vi "sCMOS_init_merFISH.vi"(4 "error in":errorcluster, 5 "Start acquisition":bool, 6 "N Frames":i32, 7 "handle":u32) -> (0 "error out":errorcluster {"code" format="%.0x"})   [LabVIEW 2015]
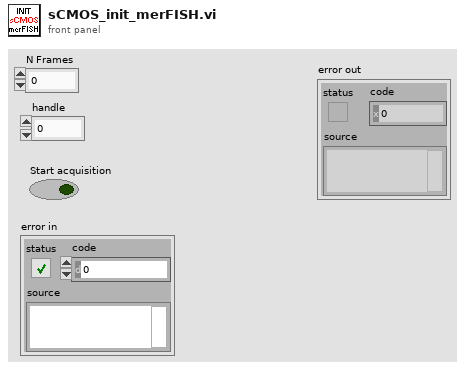
[diagram p1: front panel]
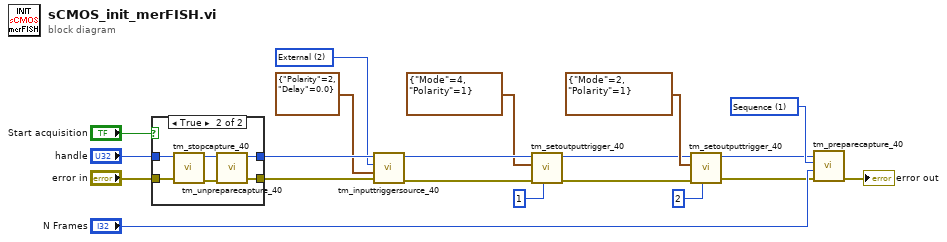
[diagram p0: block diagram]
diagram:
  w12 = 2 items=["Internal"=1, "External"=2, "Software"=3, "Master Pulse"=4] ("Source")
  w15 = 1 items=["Snap", "Sequence"] ("Capture mode")
  n1 = case shown="True" "Start acquisition" {
    tunnel: "error in" -> [w22 w28]
    tunnel: [w22 w24] -> w13
    tunnel: "handle" -> [w21 w27]
    tunnel: [w21 w23] -> w14
    frame False {
    }
    frame True {
      n2 = call <userlib>:"tm_stopcapture_40.vi"("error in (no error)"=w28, "Handle in"=w27) -> ("error out"=w26:errorcluster, "Handle out"=w25:u32)  [unwired: 8 in]
      n3 = call <userlib>:"tm_unpreparecapture_40.vi"("error in (no error)"=w26, "Handle in"=w25) -> ("error out"=w24:errorcluster, "Handle out"=w23:u32)  [unwired: 8 in]
    }
  }
  n4 = call <userlib>:"tm_inputtriggersource_40.vi"("error in (no error)"=w13, "External Options"=cluster{"Polarity":i32, "Delay":dbl} {"Polarity"=2, "Delay"=0.0}, "Source"=w12, "Handle in"=w14) -> ("error out"=w9:errorcluster, "Handle out"=w10:u32)  [unwired: 6 in]
  n5 = call <userlib>:"tm_setoutputtrigger_40.vi"("Port"=1, "error in (no error)"=w9, "Type"=cluster{"Mode":u32, "Polarity":u32} {"Mode"=4, "Polarity"=1}, "Handle in"=w10) -> ("error out"=w3:errorcluster, "Handle out"=w4:u32)  [unwired: 6 in]
  n6 = call <userlib>:"tm_setoutputtrigger_40.vi"("Port"=2, "error in (no error)"=w3, "Type"=cluster{"Mode":u32, "Polarity":u32} {"Mode"=2, "Polarity"=1}, "Handle in"=w4) -> ("error out"=w1:errorcluster, "Handle out"=w2:u32)  [unwired: 6 in]
  n7 = call <userlib>:"tm_preparecapture_40.vi"("error in (no error)"=w1, "Frames"="N Frames", "Capture mode"=w15, "Handle in"=w2) -> ("error out"=→"error out":errorcluster)  [unwired: 4 in, 3 out]
